vi "Power_Open.vi"(8 "error in (no error)":errorcluster, 9 "Port":u16 caption="Port:", 11 "IP:":string) -> (0 "error out":errorcluster, 1 "Connected?":bool, 3 "connection ID":refnum<k5>)   [LabVIEW 2020]
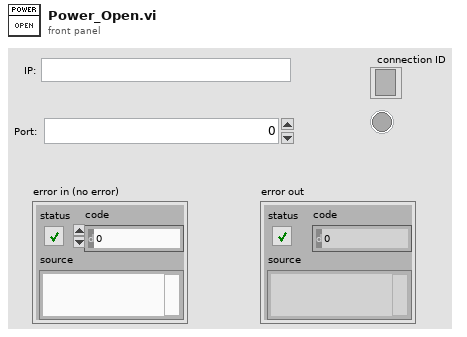
[diagram p1: front panel]
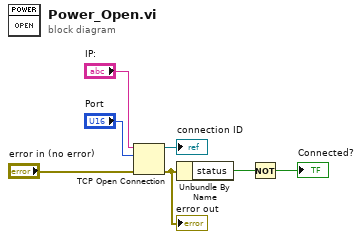
[diagram p0: block diagram]
diagram:
  n1 = TCP Open Connection(address="IP:", remote port or service name="Port", error in (no error)="error in (no error)") -> (connection ID=→"connection ID":refnum<k5>, error out=w5:errorcluster)  [unwired: 2 in]
  "error out" <- w5
  n2 = Unbundle By Name(w5) -> ("status"=w4:bool)
  n3 = Not(x=w4) -> (.not. x?=→"Connected?":bool)
